vi "Get Queue From Registry.vi"(0 "name":string, 11 "error in":errorcluster) -> (4 "queue out":T1, 15 "error out":errorcluster)   [LabVIEW 2015, in "TLB` Template.lvlib" / "AMC.lvlib"]
doc: "Returns the queue reference for the specified message queue name if it exists.\n\nThis VI returns an error if the message queue cannot be found in the queue registry.TLB Prime - Application Template 1.3.0.24\nNorm Kirchner, NI Systems Engineering - NI\nCopyright (c) 2014, NI"
uses:
  AMC.lvlib
  Message Queue.ctl
  Message.ctl
  Tools/Keyed Array/KeyedArray.ctl
  Queue Registry Method.ctl
  Queue Registry Properties.ctl
  Tools/Keyed Array/Tools_KeyedArray.lvlib
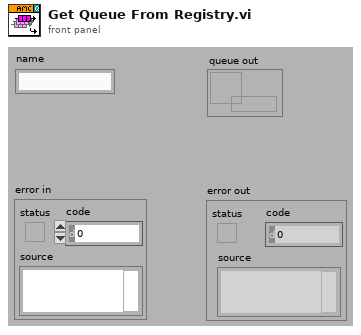
[diagram p1: front panel]
types:
  T1 = typedef "TLB` Template.lvlib/AMC.lvlib/Message Queue.ctl" = refnum<queue>
  T2 = typedef "TLB` Template.lvlib/AMC.lvlib/Queue Registry Properties.ctl" = cluster{"Name":string}
  T3 = typedef "TLB` Template.lvlib/AMC.lvlib/Queue Registry Method.ctl" = enum16{"Initialize", "Add Queue", "Set Properties", "Get Queue by Index", "Get Queue by Name", "Remove Queue", "Remove All Queues"}
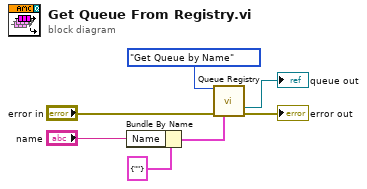
[diagram p0: block diagram]
diagram:
  n1 = Bundle By Name(cluster=T2 {"Name"=""} ("Properties In"), "Name"="name") -> (w4:T2)
  n2 = call "Queue Registry.vi"("method"=Queue_Registry_Method."Get Queue by Name" ("Method"), "error in"="error in", "properties in"=w4) -> ("message queue out"=→"queue out":T1, "error out"=→"error out":errorcluster)  [unwired: 7 in, 4 out]
